vi "7 dèn vòng lặp.vi"() -> ()   [LabVIEW 2020]
panel:
  in  "stop":bool
  out "7":bool
  out "6":bool
  out "5":bool
  out "4":bool
  out "3":bool
  out "2":bool
  out "1":bool
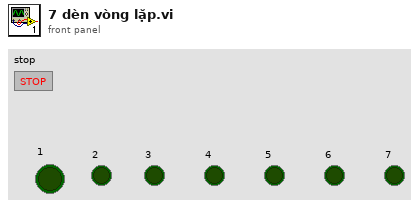
[diagram p1: front panel]
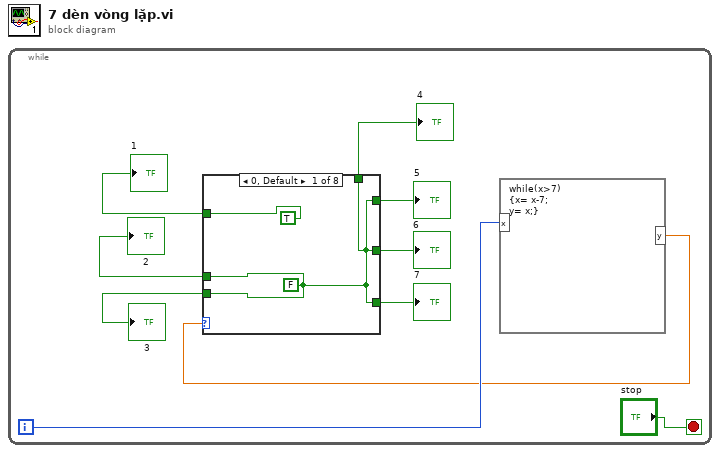
[diagram p0: block diagram]
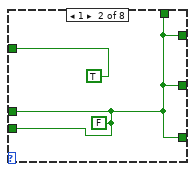
[diagram p2: hidden frame]
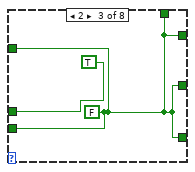
[diagram p3: hidden frame]
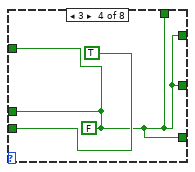
[diagram p4: hidden frame]
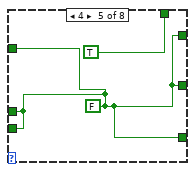
[diagram p5: hidden frame]
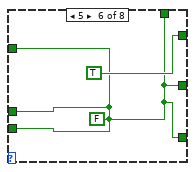
[diagram p6: hidden frame]
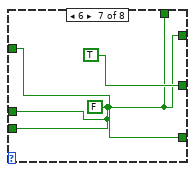
[diagram p7: hidden frame]
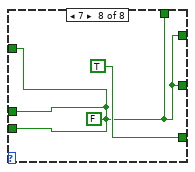
[diagram p8: hidden frame]
diagram:
  n1 = while {
    i -> [w10]
    stop <- "stop" stop-if-true
    n2 = formula code="while(x>7)\n{x= x-7;\ny= x;}"("x"=w10) -> ("y"=w9:dbl)
    n3 = case shown="0, Default" w9 {
      tunnel: [TRUE TRUE w15 w17 w19 w21 w23 w25] -> w7
      tunnel: [w11 w13 TRUE w17 w19 w21 w23 w25] -> w6
      tunnel: [w11 w13 w15 TRUE w19 w21 w23 w25] -> w5
      tunnel: [w11 w13 w15 w17 TRUE w21 w23 w25] -> w4
      tunnel: [w11 w13 w15 w17 w19 TRUE w23 w25] -> w3
      tunnel: [w11 w13 w15 w17 w19 w21 TRUE w25] -> w2
      tunnel: [w11 w13 w15 w17 w19 w21 w23 TRUE] -> w1
      frame 0, Default {
        w11 = FALSE
      }
      frame 1 {
        w13 = FALSE
      }
      frame 2 {
        w15 = FALSE
      }
      frame 3 {
        w17 = FALSE
      }
      frame 4 {
        w19 = FALSE
      }
      frame 5 {
        w21 = FALSE
      }
      frame 6 {
        w23 = FALSE
      }
      frame 7 {
        w25 = FALSE
      }
    }
    "1" <- w7
    "2" <- w6
    "3" <- w5
    "4" <- w4
    "5" <- w3
    "6" <- w2
    "7" <- w1
  }
